vi "BRig_RT__Case_Exp__UploadClosedLoop_parse.vi"(11 "input_strCmd":string) -> (0 "output_val":u16, 1 "output_idx":i32, 2 "output_dataType":u8, 3 "output_haveCmd":bool)   [LabVIEW 2014]
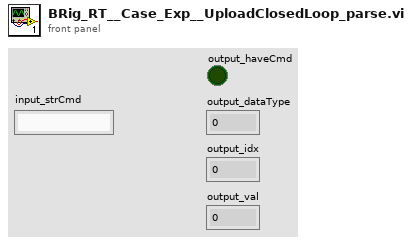
[diagram p1: front panel]
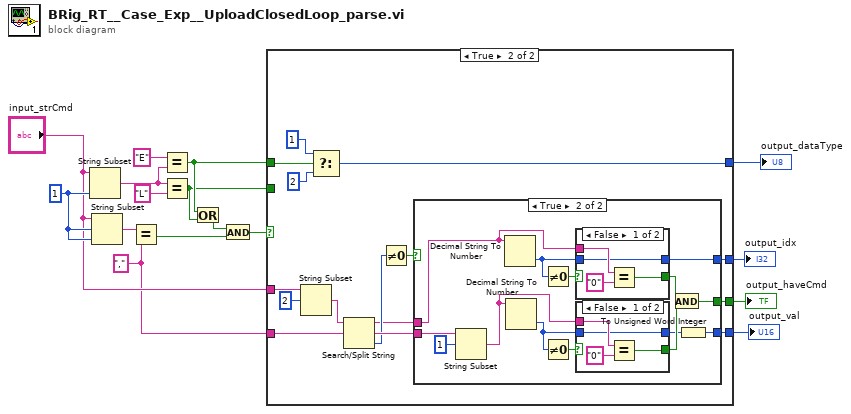
[diagram p0: block diagram]
diagram:
  w5 = "," ("y")
  w16 = 1 ("length (rest)")
  n1 = String Subset(string="input_strCmd", length (rest)=w16) -> (substring=w14:string)  [unwired: 1 in]
  n2 = String Subset(string="input_strCmd", offset (0)=w16, length (rest)=w16) -> (substring=w15:string)
  n3 = Equal?(x=w15, y=w5) -> (x = y?=w10:bool)
  n4 = Equal?(x="E", y=w14) -> (x = y?=w8:bool)
  n5 = Equal?(x=w14, y="L") -> (x = y?=w7:bool)
  n6 = Or(x=w8, y=w7) -> (x .or. y?=w11:bool)
  n7 = And(x=w11, y=w10) -> (x .and. y?=w9:bool)
  n8 = case shown="True" w9 {
    tunnel: w8 -> [_ w31]
    tunnel: w7 -> [_ _]
    tunnel: "input_strCmd" -> [_ w28]
    tunnel: w5 -> [_ w25]
    tunnel: [_ w23] -> w4
    tunnel: [_ w19] -> w1
    tunnel: [_ w18] -> w2
    tunnel: [_ w17] -> w3
    frame False {
    }
    frame True {
      n9 = String Subset(string=w28, offset (0)=2) -> (substring=w26:string)  [unwired: 1 in]
      n10 = Select(t=u8 1 ("length (rest)"), s=w31, f=u8 2 ("length (rest)")) -> (s? t:f=w23:u8)
      n11 = Search/Split String(string=w26, search string/char (-)=w25) -> (substring before match=w20:string, match + rest of string=w24:string, offset of match=w22:i32)  [unwired: 1 in]
      n12 = Not Equal To 0?(x=w22) -> (x != 0?=w21:bool)
      n13 = case shown="True" w21 {
        tunnel: w24 -> [_ w44]
        tunnel: w20 -> [_ w41]
        tunnel: [_ w33] -> w19
        tunnel: [_ w32] -> w18
        tunnel: [_ w35] -> w17
        frame False {
        }
        frame True {
          n14 = String Subset(string=w44, offset (0)=1) -> (substring=w38:string)  [unwired: 1 in]
          n15 = Decimal String To Number(string=w41) -> (number=w42:i32)  [unwired: 2 in, 1 out]
          n16 = Decimal String To Number(string=w38) -> (number=w39:i32)  [unwired: 2 in, 1 out]
          n17 = Not Equal To 0?(x=w42) -> (x != 0?=w43:bool)
          n18 = Not Equal To 0?(x=w39) -> (x != 0?=w40:bool)
          n19 = case shown="False" w43 {
            selector: w43 -> [_ w57]
            tunnel: w42 -> [w52 w56]
            tunnel: w41 -> [w55 _]
            tunnel: [w53 w57] -> w37
            tunnel: [w52 w56] -> w32
            frame False {
              n20 = Equal?(x=w55, y="0") -> (x = y?=w53:bool)
            }
            frame True {
            }
          }
          n21 = case shown="False" w40 {
            selector: w40 -> [_ w51]
            tunnel: w39 -> [w46 w50]
            tunnel: w38 -> [w49 _]
            tunnel: [w47 w51] -> w36
            tunnel: [w46 w50] -> w34
            frame False {
              n22 = Equal?(x=w49, y="0") -> (x = y?=w47:bool)
            }
            frame True {
            }
          }
          n23 = And(x=w37, y=w36) -> (x .and. y?=w35:bool)
          n24 = To Unsigned Word Integer(number=w34) -> (unsigned 16bit integer=w33:u16)
        }
      }
    }
  }
  "output_dataType" <- w4
  "output_haveCmd" <- w3
  "output_idx" <- w2
  "output_val" <- w1
